vi "DataToDB_Testing.vi"(8 "error in (no error)":errorcluster, 9 "all string":string, 10 "Procedure name":string, 11 "DSN name":string) -> (0 "error out":errorcluster, 3 "ReportStrA":string)   [LabVIEW 2013]
uses:
  <vilib>/addons/database/Connection.llb/DB Tools Open Connec (String).vi
  <vilib>/addons/database/Connection.llb/Conn Execute.vi
  <vilib>/addons/database/Recordset.llb/Rec Fetch Recordset Data (R).vi
  <vilib>/addons/database/Recordset.llb/Rec Destroy - Connection.vi
  <vilib>/addons/database/NI_Database_API.lvlib
panel:
  out "连接的字符串":string
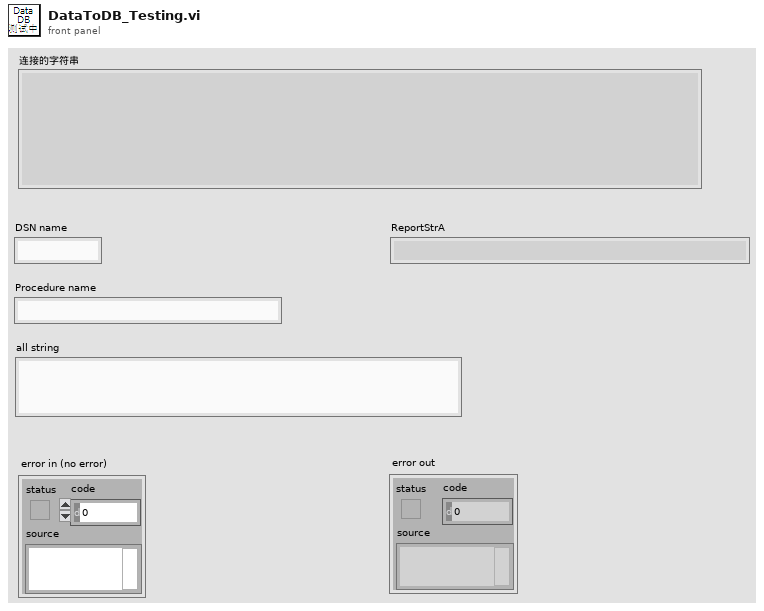
[diagram p1: front panel]
types:
  T1 = typedef "NI_Database_API.lvlib/Conn ObjectReference.ctl" = refnum<k1>
  T2 = typedef "NI_Database_API.lvlib/Rec ObjectReference.ctl" = refnum<k1>
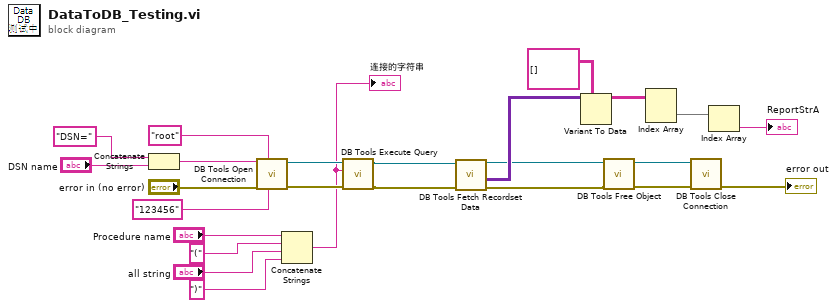
[diagram p0: block diagram]
diagram:
  n1 = Concatenate Strings("DSN=", "DSN name") -> (w15:string)
  n2 = call-poly <vilib>:"DB Tools Open Connection.vi"("password"="123456" ("userID"), "userID"="root", "error in (no error)"="error in (no error)", "connection information"=w15) -> ("error out"=w25:errorcluster, "connection reference"=w24:T1)  [unwired: 4 in]
  n3 = Concatenate Strings("Procedure name", "(", "all string", ")") -> (w20:string)
  "连接的字符串" <- w20
  n4 = call-poly <vilib>:"DB Tools Execute Query.vi"("error in (no error)"=w25, "SQL query"=w20, "connection reference"=w24) -> ("error out"=w8:errorcluster, "recordset reference"=w9:T2)  [unwired: 5 in]
  n5 = call-poly <vilib>:"DB Tools Fetch Recordset Data.vi"("error in (no error)"=w8, "recordset reference"=w9) -> ("error out"=w6:errorcluster, "recordset data"=w11:variant[][], "recordset reference out"=w7:T2)  [unwired: 3 in]
  n6 = Variant To Data(type=string[][] [], Variant=w11) -> (data=w5:string[][])  [unwired: 1 in, 1 out]
  n7 = call-poly <vilib>:"DB Tools Free Object.vi"("error in (no error)"=w6, "recordset reference"=w7) -> ("error out"=w22:errorcluster, "connection reference"=w23:T1)  [unwired: 8 in]
  n8 = Index Array(array=w5) -> (element=w4:string[])  [unwired: 2 in]
  n9 = call <vilib>:"DB Tools Close Connection.vi"("error in (no error)"=w22, "connection reference"=w23) -> ("error out"=→"error out":errorcluster)  [unwired: 5 in]
  n10 = Index Array(array=w4) -> (element=→"ReportStrA":string)  [unwired: 1 in]
